vi "Create DMM Tags.vi"(8 "error in (no error)":errorcluster, 11 "CVT Tags to Create":T1) -> (0 "error out":errorcluster, 3 "CVT Tags to Create":T1)   [LabVIEW 2016, in "CVT.lvlib"]
uses:
  CVT.lvlib
  Support Libraries/Current Value Table/Type Defs/File Format.ctl
  Support Libraries/Current Value Table/Type Defs/Single Tag.ctl
  Support Libraries/Current Value Table/Type Defs/Data Types.ctl
  Support Libraries/Current Value Table/Type Defs/Tag Grouping set.ctl
  Support Libraries/Current Value Table/Current Value Table.lvlib
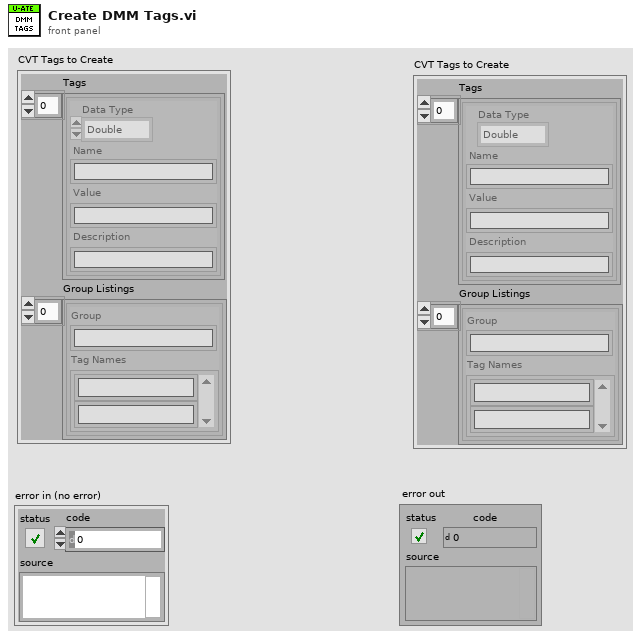
[diagram p1: front panel]
types:
  T1 = typedef "CVT.lvlib/Current Value Table.lvlib/File Format.ctl" = cluster{"Tags":T2[], "Group Listings":T4[]}
  T2 = typedef "CVT.lvlib/Current Value Table.lvlib/Single Tag.ctl" = cluster{"Data Type":T3, "Name":string, "Value":string, "Description":string}
  T3 = typedef "CVT.lvlib/Current Value Table.lvlib/Data Types.ctl" = enum16{"Double", "Single", "I64", "I32", "I16", "I8", "U64", "U32", "U16", "U8", "String", "Boolean", "Array of U8", "Array of U16", "Array of U32", "Array of U64", "Array of I64", "Array of I32", "Array of I16", "Array of I8", "Array of Double", "Array of Single", "Array of Boolean", "Array of String"}
  T4 = typedef "CVT.lvlib/Current Value Table.lvlib/Tag Grouping set.ctl" = cluster{"Group":string, "Tag Names":string[]}
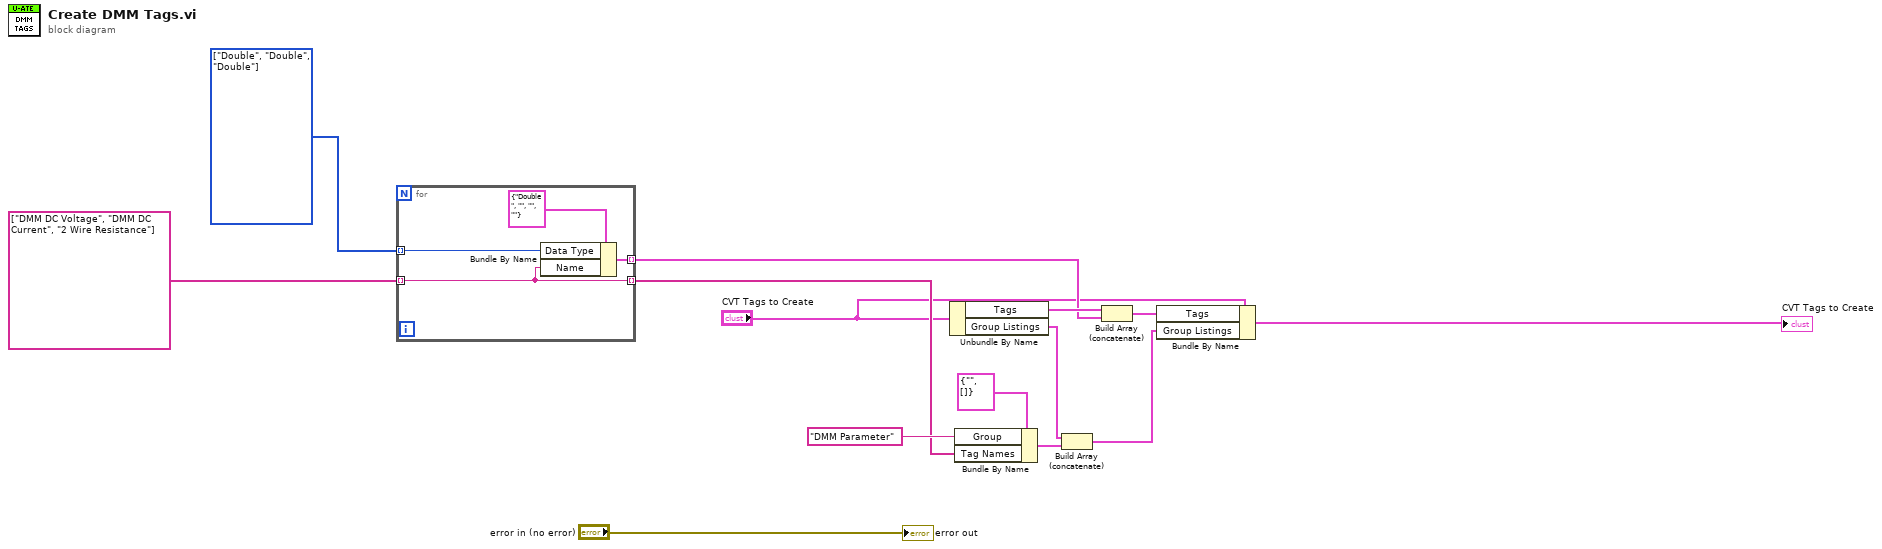
[diagram p0: block diagram]
diagram:
  w4 = T3[] [enum."Double", enum."Double", enum."Double"] items=["Double", "Single", "I64", "I32", "I16", "I8", "U64", "U32", "U16", "U8", "String", "Boolean", "Array of U8", "Array of U16", "Array of U32", "Array of U64", "Array of I64", "Array of I32", "Array of I16", "Array of I8", "Array of Double", "Array of Single", "Array of Boolean", "Array of String"] ("Array")
  n1 = for {
    tunnel: string[] ["DMM DC Voltage", "DMM DC Current", "2 Wire Resistance"] -> [w17] mode=indexing
    tunnel: [w18] -> w13 mode=indexing
    tunnel: [w17] -> w10 mode=indexing
    tunnel: w4 -> [w15] mode=indexing
    n2 = Bundle By Name(cluster=T2 {"Data Type"=enum."Double", "Name"="", "Value"="", "Description"=""} ("element"), "Data Type"=w15, "Name"=w17) -> (w18:T2)
  }
  n3 = Unbundle By Name("CVT Tags to Create") -> ("Tags"=w14:T2[], "Group Listings"=w9:T4[])
  n4 = Bundle By Name(cluster=T4 {"Group"="", "Tag Names"=[]} ("Tag Grouping"), "Group"="DMM Parameter", "Tag Names"=w10) -> (w8:T4)
  n5 = Build Array (concatenate)(w9, w8) -> (w7:T4[])
  n6 = Build Array (concatenate)(w14, w13) -> (w12:T2[])
  n7 = Bundle By Name(cluster="CVT Tags to Create", "Tags"=w12, "Group Listings"=w7) -> (→"CVT Tags to Create":T1)
  "error out" <- "error in (no error)"
